vi "Configure Measurement (Demodulation - AM or FM ).vi"(0 "VISA resource name":refnum<visa-resource-name>, 1 "Enable Peak Hold State (F: Disable)":bool, 2 "IF Bandwidth (0: 1.2MHz)":i32(ring) items=["1.2MHz", "960Hz", "600Hz", "480Hz", "300Hz", "240Hz", "120Hz", "96Hz", "60Hz"], 5 "Enable Averaging (F: Disable)":bool, 7 "Average Count (10)":dbl=10.0, 9 "Detector Type (0: Positive Peak)":i32(ring) items=["Positive Peak", "Negative Peak", "Average Peak", "RMS"], 11 "error in (no error)":errorcluster, 12 "Equal Low Pass Filter (0: Auto)":i32(ring) items=["Auto", "Off", "IFBW6", "IFBW20", "IFBW60", "IFBW200", "IFBW600", "IFBW2000"], 13 "Auto IF Bandwidth (F: Disable)":bool) -> (4 "VISA resource name out":refnum<visa-resource-name>, 15 "error out":errorcluster)   [LabVIEW 2022 SP3, in "Agilent N934X Series.lvlib"]
doc: "Configures the general setting for AM or FM demodulation of Demodulation Option.\n\nNote:\nThis VI is only applicable for N9321C, N9322C, N9323C, N9324C models"
uses:
  <instrlib>/Agilent N934X Series/Agilent N934X Series.lvlib
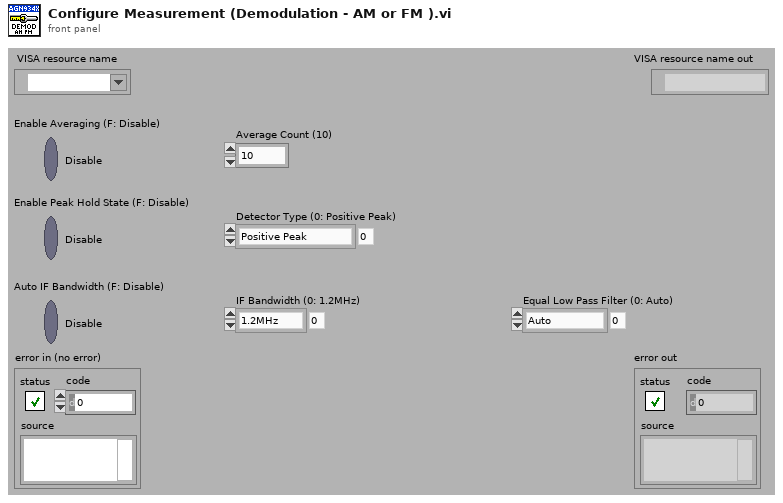
[diagram p1: front panel]
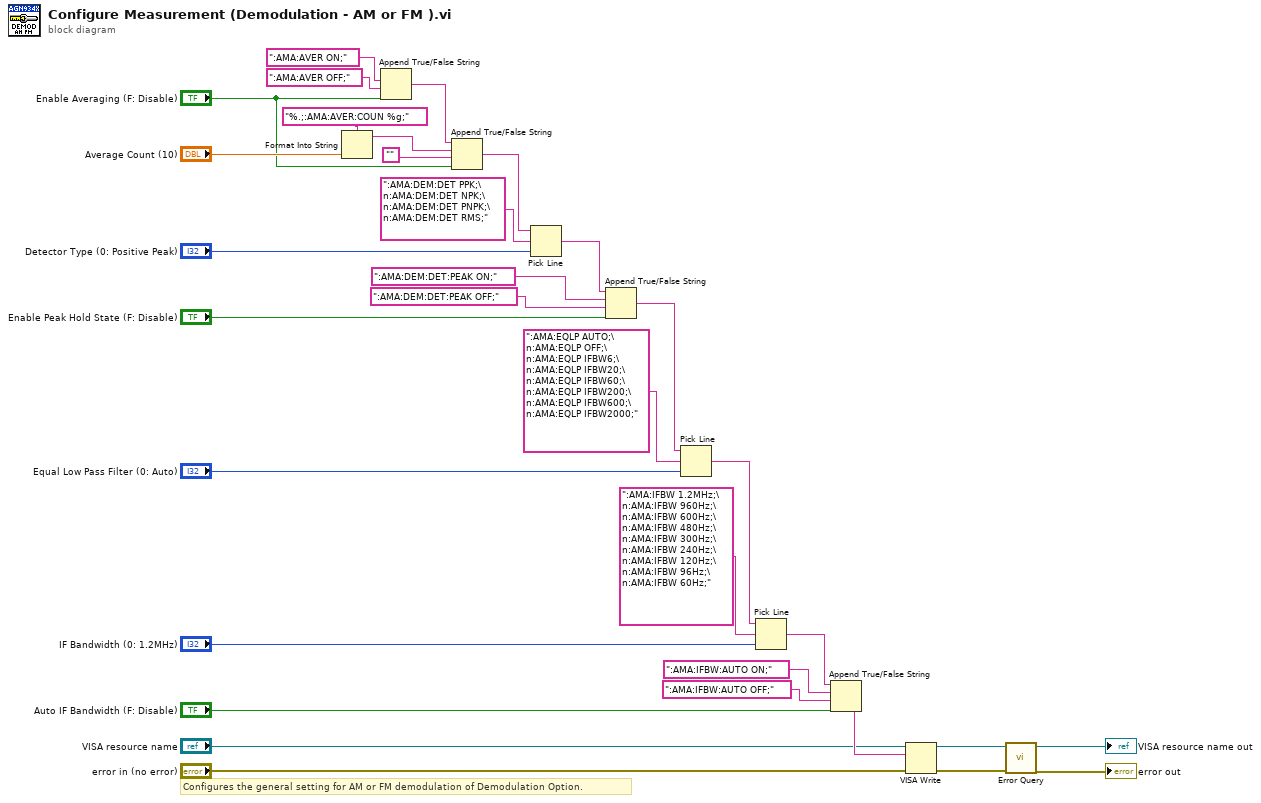
[diagram p0: block diagram]
diagram:
  # "Configures the general setting for AM or FM demodulation of Demodulation Option."
  n1 = Format Into String(format string="%.;:AMA:AVER:COUN %g;", "Average Count (10)") -> (resulting string=w3:string)  [unwired: 2 in, 1 out]
  n2 = Append True/False String(1:"Enable Averaging (F: Disable)", 2:":AMA:AVER OFF;", 3:":AMA:AVER ON;") -> (0:w4:string)  [unwired: 1 in]
  n3 = Append True/False String(1:"Enable Averaging (F: Disable)", 2:"", 3:w3, 4:w4) -> (0:w1:string)
  n4 = Pick Line(string ("")=w1, multi-line string=":AMA:DEM:DET PPK;\n:AMA:DEM:DET NPK;\n:AMA:DEM:DET PNPK;\n:AMA:DEM:DET RMS;", line index="Detector Type (0: Positive Peak)") -> (output string=w26:string)
  n5 = Append True/False String(1:"Enable Peak Hold State (F: Disable)", 2:":AMA:DEM:DET:PEAK OFF;", 3:":AMA:DEM:DET:PEAK ON;", 4:w26) -> (0:w20:string)
  n6 = Pick Line(string ("")=w20, multi-line string=":AMA:EQLP AUTO;\n:AMA:EQLP OFF;\n:AMA:EQLP IFBW6;\n:AMA:EQLP IFBW20;\n:AMA:EQLP IFBW60;\n:AMA:EQLP IFBW200;\n:AMA:EQLP IFBW600;\n:AMA:EQLP IFBW2000;", line index="Equal Low Pass Filter (0: Auto)") -> (output string=w17:string)
  n7 = Pick Line(string ("")=w17, multi-line string=":AMA:IFBW 1.2MHz;\n:AMA:IFBW 960Hz;\n:AMA:IFBW 600Hz;\n:AMA:IFBW 480Hz;\n:AMA:IFBW 300Hz;\n:AMA:IFBW 240Hz;\n:AMA:IFBW 120Hz;\n:AMA:IFBW 96Hz;\n:AMA:IFBW 60Hz;", line index="IF Bandwidth (0: 1.2MHz)") -> (output string=w16:string)
  n8 = Append True/False String(1:"Auto IF Bandwidth (F: Disable)", 2:":AMA:IFBW:AUTO OFF;", 3:":AMA:IFBW:AUTO ON;", 4:w16) -> (0:w12:string)
  n9 = VISA Write(VISA resource name="VISA resource name", write buffer=w12, error in (no error)="error in (no error)") -> (VISA resource name out=w9:refnum<visa-resource-name>, error out=w8:errorcluster)  [unwired: 1 out]
  n10 = call <instrlib>:"Error Query.vi"("error in (no error)"=w8, "VISA resource name"=w9) -> ("error out"=→"error out":errorcluster, "VISA resource name out"=→"VISA resource name out":refnum<visa-resource-name>)  [unwired: 6 in, 2 out]
